vi "Angle Stat (SubVI).vi"(9 "Angle Valid":bool, 10 "Angle":fxp<+/-,16,3> format="%.14g", 11 "Done In":bool) -> (0 "Mean Angle":fxp<+/-,32,16> format="%.14g", 1 "Min Angle":fxp<+/-,16,3> format="%.14g", 2 "Max Angle":fxp<+/-,16,3> format="%.14g", 3 "Done Out":bool)   [LabVIEW 2015]
uses:
  <vilib>/rvi/FXPMathLib/FxpDiv/subVIs/nifxpmath_Div_SimConfig.ctl
  <vilib>/rvi/FXPMathLib/FxpDiv/simVIs/DllFxpDivTemp_sub.vi
  <vilib>/rvi/FXPMathLib/FxpDiv/XNode/nifxpmath_Div.xnode
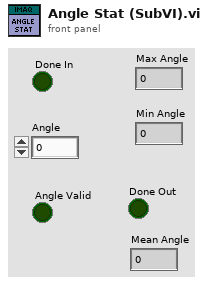
[diagram p1: front panel]
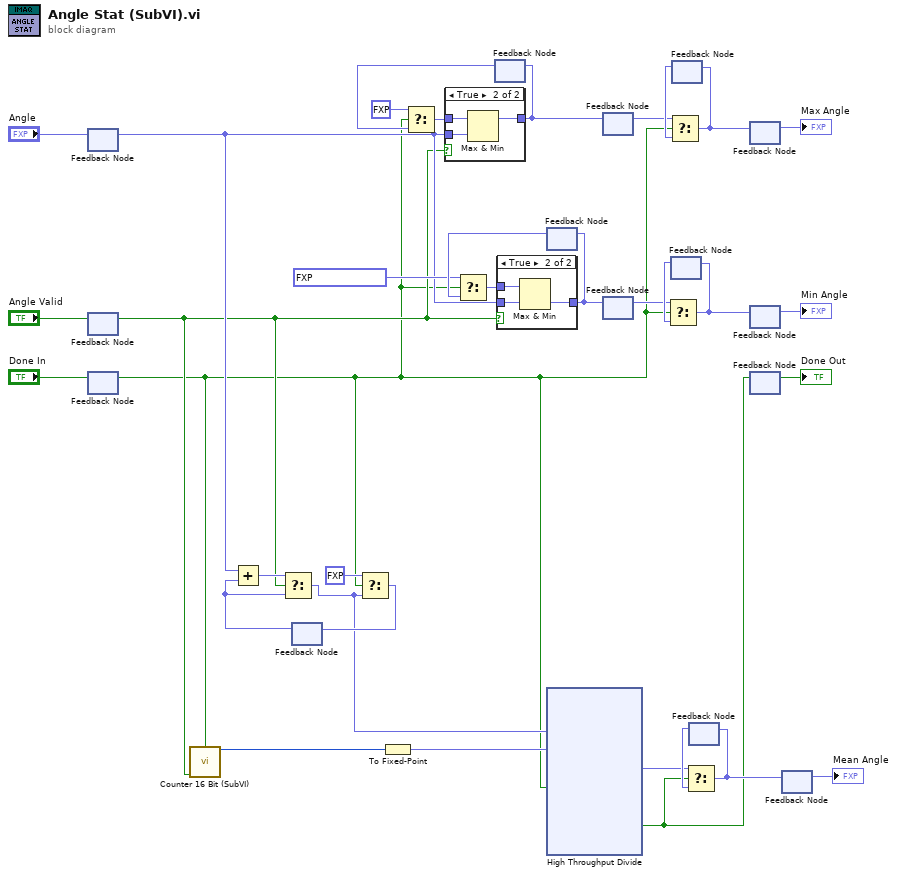
[diagram p0: block diagram]
diagram:
  n1 = feedback-in #1("Angle") -> ()
  n2 = feedback #1() -> (w15:fxp<+/-,16,3>)  [unwired: 1 in]
  n3 = feedback-in #2("Angle Valid") -> ()
  n4 = feedback #2() -> (w10:bool)  [unwired: 1 in]
  n5 = feedback-in #3("Done In") -> ()
  n6 = feedback #3() -> (w6:bool)  [unwired: 1 in]
  n7 = call "Counter 16 Bit (SubVI).vi"("RESET"=w6, "Enable"=w10) -> ("Count"=w8:u16)  [unwired: 11 in, 2 out]
  n8 = feedback #4() -> (w11:fxp<+/-,32,16>)  [unwired: 1 in]
  n9 = Add(x=w15, y=w11) -> (x+y=w12:fxp<+/-,32,16>)
  n10 = Select(t=w12, s=w10, f=w11) -> (s? t:f=w9:fxp<+/-,32,16>)
  n11 = Select(t=fxp<+/-,32,16> 0.0, s=w6, f=w9) -> (s? t:f=w14:fxp<+/-,32,16>)
  n12 = feedback-in #4(w14) -> ()
  n13 = To Fixed-Point(number=w8) -> (fixed-point=w7:fxp<+/-,16,16>)  [unwired: 1 in]
  n14 = feedback #5() -> (w17:fxp<+/-,16,3>)  [unwired: 1 in]
  n15 = Select(t=fxp<+/-,16,3> 0.0, s=w6, f=w17) -> (s? t:f=w18:fxp<+/-,16,3>)
  n16 = case shown="True" w10 {
    tunnel: w15 -> [_ w39]
    tunnel: [w36 w38] -> w24
    tunnel: w18 -> [w36 w37]
    frame False {
    }
    frame True {
      n17 = Max & Min(x=w37, y=w39) -> (max(x,y)=w38:fxp<+/-,16,3>)  [unwired: 1 out]
    }
  }
  n18 = feedback-in #5(w24) -> ()
  n19 = feedback #6() -> (w22:fxp<+/-,16,3>)  [unwired: 1 in]
  n20 = Select(t=fxp<+/-,16,3> 3.9998779296875, s=w6, f=w22) -> (s? t:f=w21:fxp<+/-,16,3>)
  n21 = case shown="True" w10 {
    tunnel: w15 -> [_ w43]
    tunnel: [w40 w41] -> w23
    tunnel: w21 -> [w40 w42]
    frame False {
    }
    frame True {
      n22 = Max & Min(x=w42, y=w43) -> (min(x,y)=w41:fxp<+/-,16,3>)  [unwired: 1 out]
    }
  }
  n23 = feedback-in #6(w23) -> ()
  n24 = xnode "High Throughput Divide"("x"=w9, "y"=w7, "input valid"=w6) -> ("x/y"=w3:fxp<+/-,32,16>, "output valid"=w1:bool)  [unwired: 1 in, 1 out]
  n25 = feedback #7() -> (w25:fxp<+/-,16,3>)  [unwired: 1 in]
  n26 = feedback-in #7(w24) -> ()
  n27 = feedback #8() -> (w26:fxp<+/-,16,3>)  [unwired: 1 in]
  n28 = feedback-in #8(w23) -> ()
  n29 = feedback #9() -> (w29:fxp<+/-,16,3>)  [unwired: 1 in]
  n30 = Select(t=w26, s=w6, f=w29) -> (s? t:f=w32:fxp<+/-,16,3>)
  n31 = feedback-in #9(w32) -> ()
  n32 = feedback #10() -> (w30:fxp<+/-,16,3>)  [unwired: 1 in]
  n33 = Select(t=w25, s=w6, f=w30) -> (s? t:f=w31:fxp<+/-,16,3>)
  n34 = feedback-in #10(w31) -> ()
  n35 = feedback #11() -> (w4:fxp<+/-,32,16>)  [unwired: 1 in]
  n36 = Select(t=w3, s=w1, f=w4) -> (s? t:f=w2:fxp<+/-,32,16>)
  n37 = feedback-in #11(w2) -> ()
  n38 = feedback #12() -> (→"Max Angle":fxp<+/-,16,3>)  [unwired: 1 in]
  n39 = feedback-in #12(w31) -> ()
  n40 = feedback #13() -> (→"Min Angle":fxp<+/-,16,3>)  [unwired: 1 in]
  n41 = feedback-in #13(w32) -> ()
  n42 = feedback #14() -> (→"Done Out":bool)  [unwired: 1 in]
  n43 = feedback-in #14(w1) -> ()
  n44 = feedback #15() -> (→"Mean Angle":fxp<+/-,32,16>)  [unwired: 1 in]
  n45 = feedback-in #15(w2) -> ()
